vi "Read Configuration Simple.vi"() -> ()   [LabVIEW 2016, in "LVOOP Introduction.lvlib"]
doc: "Illustrates how to read a configuration settings file.\n\nLizenziert unter EUPL V. 1.1"
uses:
  LVOOP Introduction.lvlib
  <vilib>/Utility/config.llb/Read Key (Boolean).vi
  <vilib>/Utility/config.llb/Read Key (Double).vi
  <vilib>/Utility/config.llb/Read Key (Path).vi
  <vilib>/Utility/config.llb/Read Key (String).vi
  <vilib>/Utility/config.llb/NI_LVConfig.lvlib
panel:
  in  "configuration file path":path
  out "Path Value":path
  out "Numeric":dbl format="%0.2f"
  out "Boolean":bool
  out "String 2":string
  out "String 1":string
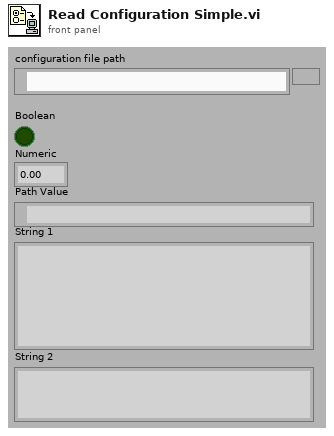
[diagram p1: front panel]
types:
  T1 = typedef "NI_LVConfig.lvlib/Config Data RefNum.ctl" = refnum<k1>
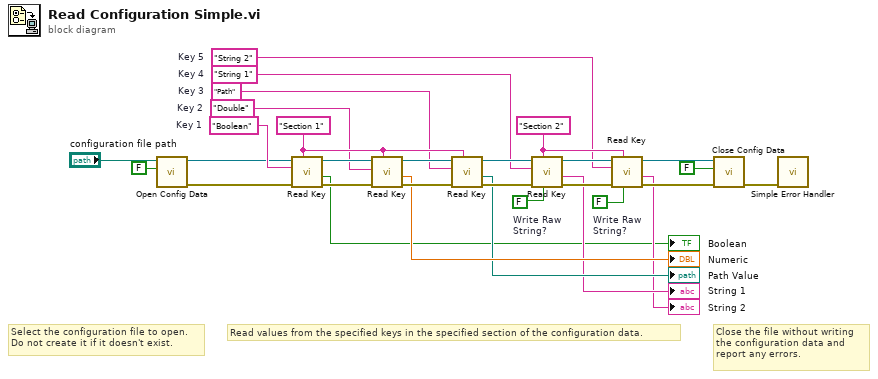
[diagram p0: block diagram]
diagram:
  w4 = FALSE  # Write Raw String?
  w5 = FALSE  # Write Raw String?
  w14 = "String 2"  # Key 5
  w15 = "String 1"  # Key 4
  w16 = "Path"  # Key 3
  w17 = "Double"  # Key 2
  w18 = "Boolean"  # Key 1
  w19 = "Section 2" ("section")
  w20 = "Section 1" ("section")
  # "Close the file without writing\nthe configuration data and\nreport any errors."
  # "Read values from the specified keys in the specified section of the configuration data."
  # "Select the configuration file to open.\nDo not create it if it doesn't exist."
  n1 = call <vilib>:"Open Config Data.vi"("create file if necessary (T)"=FALSE ("create file if necessary? (T)"), "configuration file path"="configuration file path") -> ("error out"=w12:errorcluster, "refnum"=w11:T1)  [unwired: 7 in, 1 out]
  n2 = call-poly <vilib>:"Read Key.vi"("section"=w20, "error in (no error)"=w12, "key"=w18, "refnum"=w11) -> ("error out"=w30:errorcluster, "value"=→"Boolean":bool, "refnum out"=w28:T1)  [unwired: 1 in, 4 out]
  n3 = call-poly <vilib>:"Read Key.vi"("section"=w20, "error in (no error)"=w30, "key"=w17, "refnum"=w28) -> ("error out"=w25:errorcluster, "value"=→"Numeric":dbl, "refnum out"=w26:T1)  [unwired: 1 in, 4 out]
  n4 = call-poly <vilib>:"Read Key.vi"("section"=w20, "error in (no error)"=w25, "key"=w16, "refnum"=w26) -> ("error out"=w29:errorcluster, "value"=→"Path Value":path, "refnum out"=w27:T1)  [unwired: 1 in, 4 out]
  n5 = call-poly <vilib>:"Read Key.vi"("read raw string? (F)"=w4, "section"=w19, "error in (no error)"=w29, "key"=w15, "refnum"=w27) -> ("error out"=w22:errorcluster, "value"=→"String 1":string, "refnum out"=w21:T1)  [unwired: 1 in, 3 out]
  n6 = call-poly <vilib>:"Read Key.vi"("read raw string? (F)"=w5, "section"=w19, "error in (no error)"=w22, "key"=w14, "refnum"=w21) -> ("error out"=w24:errorcluster, "value"=→"String 2":string, "refnum out"=w23:T1)  [unwired: 1 in, 3 out]
  n7 = call <vilib>:"Close Config Data.vi"("error in (no error)"=w24, "write file if changed (T)"=FALSE ("write configuration file? (T)"), "refnum"=w23) -> ("error out"=w13:errorcluster)  [unwired: 8 out]
  n8 = call <vilib>:"Simple Error Handler.vi"("error in (no error)"=w13) -> ()  [unwired: 1 in, 8 out]
